vi "getData.vi"(8 "error in (no error)":errorcluster, 10 "device_name":string, 11 "ScriptEventList in":refnum<class "ScriptEventList.lvclass">) -> (0 "error out":errorcluster, 1 "singleToneData":T2(array[cluster]), 2 "data out":T3(array[cluster]) {"time" format="%_18g"}, 3 "ScriptEventList out":refnum<class "ScriptEventList.lvclass">, 4 "dataType":T1(ring))   [LabVIEW 2011, in "Tools.lvlib" / "Scripting.lvlib" / "ScriptEventList.lvclass"]
uses:
  ScriptEventList.lvclass
  DatabaseHelpers/Database Objects/Channel/Channel.lvclass
  ScriptEventList.lvclass/ScriptEventList.ctl
  ScriptEvent.lvclass
  ScriptEvents/SingleTone/SingleTone.lvclass
panel:
  out "Array":dbl[](array[numeric]) format="%_10g"
  out "times out":dbl[](array[numeric]) format="%_10g"
  out "appended array":dbl[](array[numeric]) format="%_13g"
  out "out":dbl[](array[numeric]) format="%_18g"
  out "in":dbl[](array[numeric])
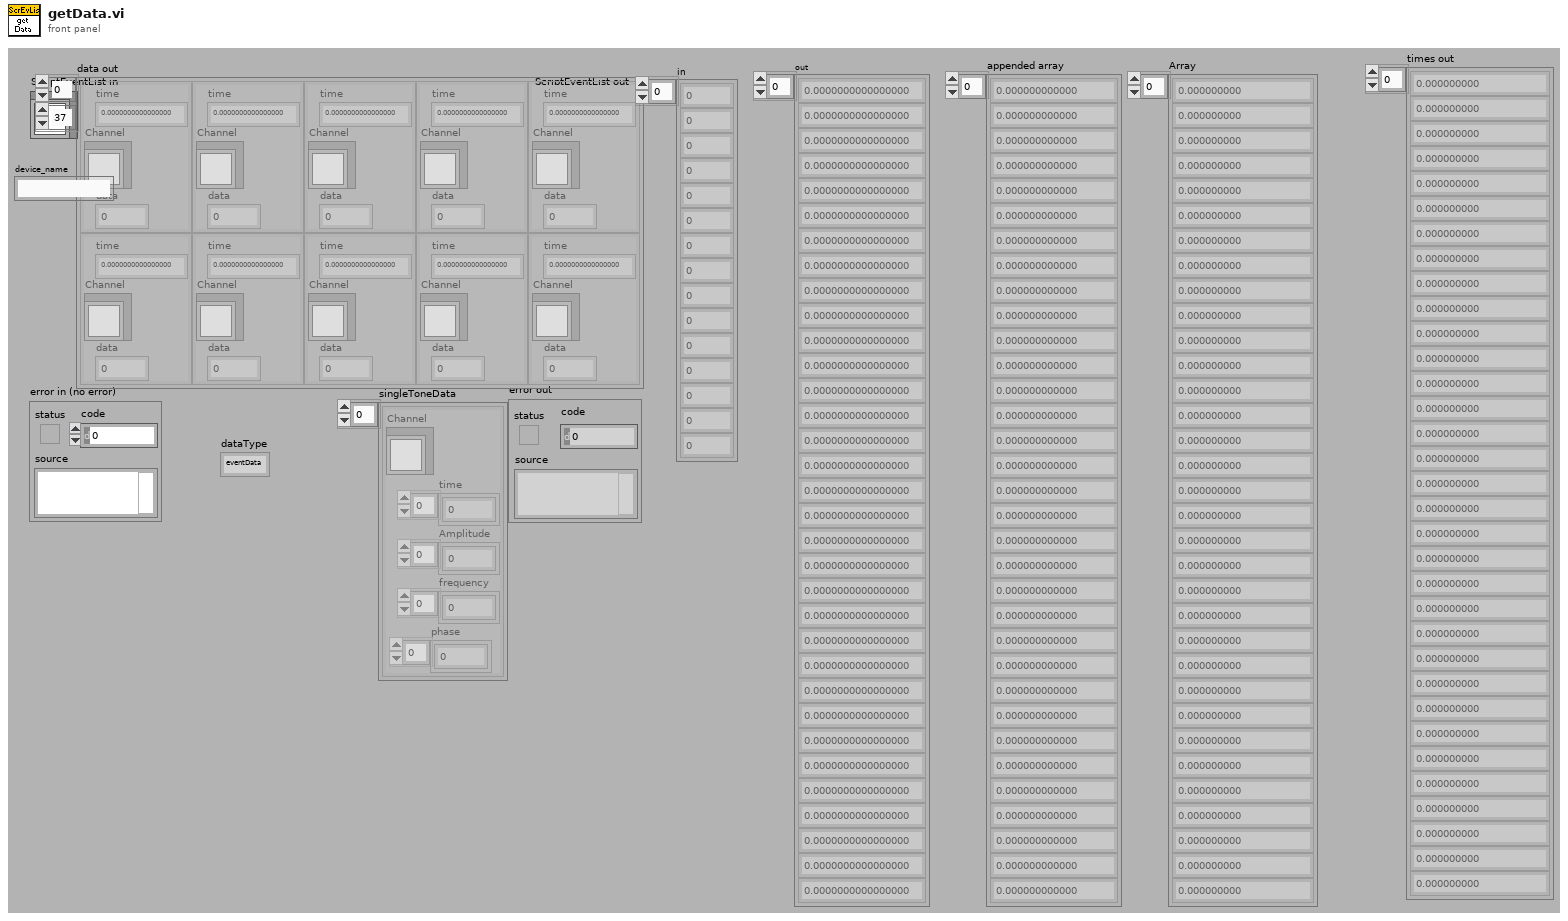
[diagram p1: front panel]
types:
  T1 = enum16{"eventData", "singleToneData", "fileData"}
  T2 = cluster{"Channel":refnum<class "Channel.lvclass">, "time":dbl[], "Amplitude":dbl[], "frequency":dbl[], "phase":dbl[]}[]
  T3 = cluster{"time":dbl, "Channel":refnum<class "Channel.lvclass">, "data":dbl}[][]
  T4 = cluster{"times":dbl[], "Channel":refnum<class "Channel.lvclass">, "data":dbl[]}
  T5 = cluster{"Tools.lvlib:DatabaseHelpers.lvlib:Channel.lvclass":refnum<class "Channel.lvclass">, "time":dbl[], "Amplitude":dbl[], "frequency":dbl[], "phase":dbl[]}[]
  T6 = cluster{dbl, "Channel":refnum<class "Channel.lvclass">, dbl}[][]
  T7 = cluster{"time":dbl, "Channel":refnum<class "Channel.lvclass">, "value":dbl}[][]
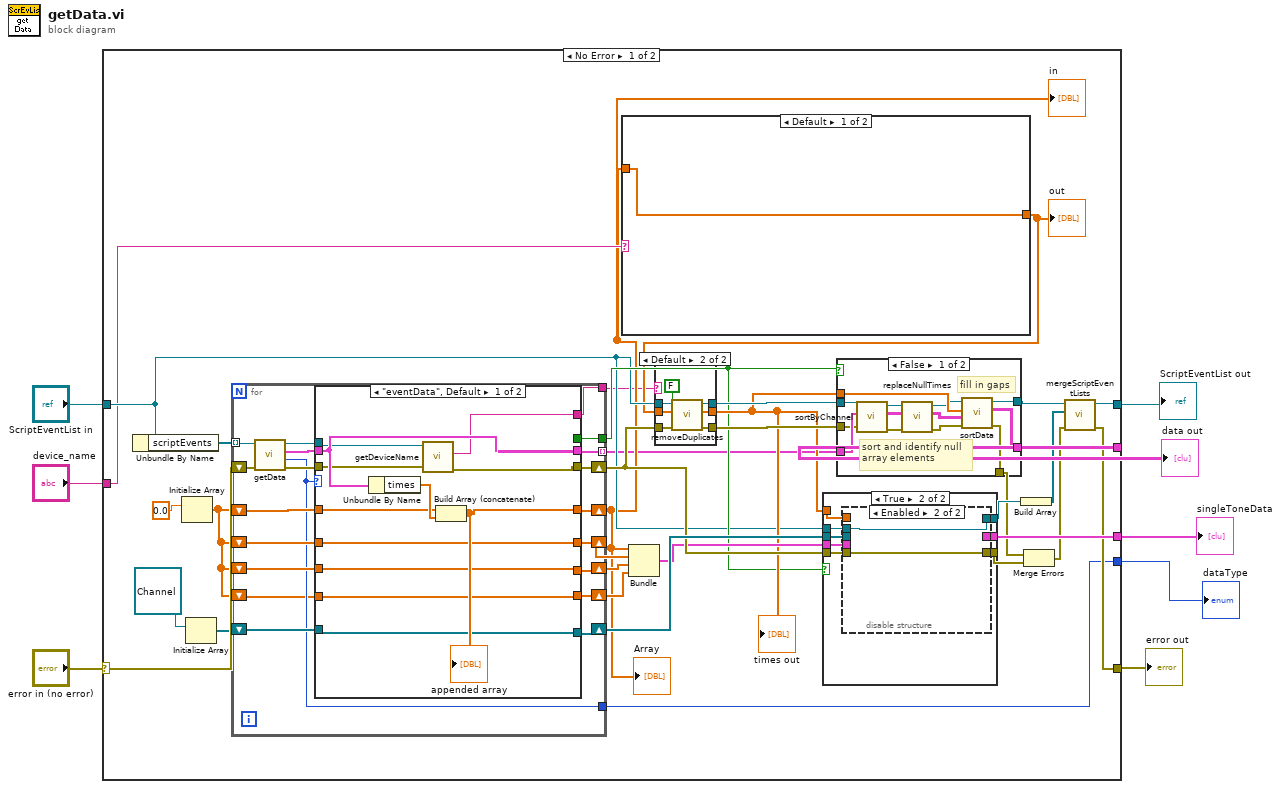
[diagram p0: block diagram]
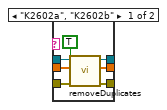
[diagram p2: hidden frame]
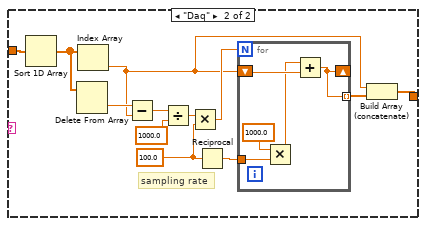
[diagram p3: hidden frame]
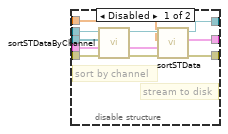
[diagram p5: hidden frame]
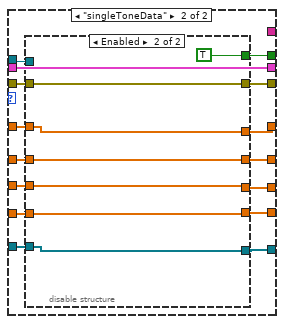
[diagram p7: hidden frame]
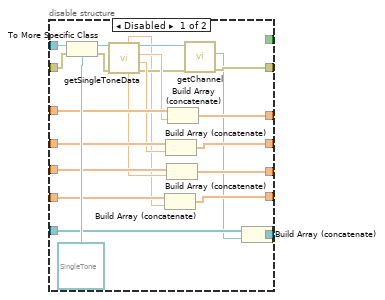
[diagram p8: hidden frame]
diagram:
  n1 = case shown="No Error" "error in (no error)" {
    selector: "error in (no error)" -> [w40 w190]
    tunnel: [w18 w190] -> w7
    tunnel: [w24 w189] -> w5
    tunnel: "ScriptEventList in" -> [w14 w189]
    tunnel: [w37 _] -> w4
    tunnel: [w27 _] -> w3
    tunnel: [w17 _] -> w2
    tunnel: "device_name" -> [w13 _]
    frame No Error {
      n2 = Unbundle By Name(w14) -> ("scriptEvents"=w41:refnum<class "ScriptEvent.lvclass">[])
      n3 = Initialize Array(0.0) -> (w16:dbl[])  [unwired: 1 in]
      n4 = Initialize Array(refnum<class "Channel.lvclass"> refnum ("Tools.lvlib:DatabaseHelpers.lvlib:Channel.lvclass")) -> (w34:refnum<class "Channel.lvclass">[])  [unwired: 1 in]
      n5 = for {
        tunnel: w41 -> [w131] mode=indexing
        shift-right: [w124] -> w31
        shift-left: w40 -> [w130]
        tunnel: [w126] -> w10 mode=indexing
        shift-right: [w128] -> w12
        shift-left: w16 -> [w129]
        shift-right: [w121] -> w33
        shift-left: w16 -> [w122]
        shift-right: [w120] -> w28
        shift-left: w16 -> [w119]
        shift-right: [w117] -> w32
        shift-left: w34 -> [w118]
        tunnel: [w116] -> w26
        tunnel: [w115] -> w17
        shift-right: [w113] -> w15
        shift-left: w16 -> [w114]
        tunnel: [w112] -> w9
        n6 = call-dynamic "getData.vi"("error in (no error)"=w130, "ScriptEvent in"=w131) -> ("error out"=w125:errorcluster, "dataType"=w115:T1, "data"=w127:T4, "ScriptEvent out"=w123:refnum<class "ScriptEvent.lvclass">)  [unwired: 6 in]
        n7 = case shown="\"eventData\", Default" w115 {
          tunnel: w129 -> [w142 w156]
          tunnel: [w141 w157] -> w128
          tunnel: w127 -> [w140 w144]
          tunnel: [w140 w144] -> w126
          tunnel: w125 -> [w134 w155]
          tunnel: [w133 w150] -> w124
          tunnel: w123 -> [w135 w158]
          tunnel: w122 -> [w139 w154]
          tunnel: [w139 w153] -> w121
          tunnel: [w138 w152] -> w120
          tunnel: w119 -> [w138 w151]
          tunnel: w118 -> [w136 w149]
          tunnel: [w136 w148] -> w117
          tunnel: [_ w147] -> w116
          tunnel: w114 -> [w137 w146]
          tunnel: [w137 w145] -> w113
          tunnel: [w132 _] -> w112
          frame "eventData", Default {
            n8 = Unbundle By Name(w140) -> ("times"=w143:dbl[])
            n9 = call "getDeviceName.vi"("error in (no error)"=w134, "ScriptEvent in"=w135) -> ("error out"=w133:errorcluster, "deviceName"=w132:string)  [unwired: 7 in, 1 out]
            n10 = Build Array (concatenate)(w142, w143) -> (w141:dbl[])
            "appended array" <- w141
          }
          frame "singleToneData" {
            n11 = disable-structure shown="Enabled" {
              disable-tunnel: w158 -> [w181 _]
              disable-tunnel: [w177 w187] -> w157
              disable-tunnel: w156 -> [w176 w187]
              disable-tunnel: w155 -> [w174 w183]
              disable-tunnel: w154 -> [w173 w186]
              disable-tunnel: [w172 w186] -> w153
              disable-tunnel: [w170 w185] -> w152
              disable-tunnel: w151 -> [w169 w185]
              disable-tunnel: [w165 w183] -> w150
              disable-tunnel: w149 -> [w164 w182]
              disable-tunnel: [w163 w182] -> w148
              disable-tunnel: [_ TRUE] -> w147
              disable-tunnel: w146 -> [w162 w184]
              disable-tunnel: [w161 w184] -> w145
              frame Disabled {
                n12 = To More Specific Class(target class=refnum<class "SingleTone.lvclass"> refnum ("Tools.lvlib:Scripting.lvlib:SingleTone.lvclass"), reference=w181, error in=w174) -> (specific class reference=w179:refnum<class "SingleTone.lvclass">, error out=w178:errorcluster)
                n13 = call "getSingleToneData.vi"("error in (no error)"=w178, "SingleTone in"=w179) -> ("error out"=w166:errorcluster, "amplitude"=w171:dbl, "time"=w175:dbl, "SingleTone out"=w167:refnum<class "SingleTone.lvclass">, "frequency"=w168:dbl, "phase"=w160:dbl)  [unwired: 4 in]
                n14 = Build Array (concatenate)(w162, w160) -> (w161:dbl[])
                n15 = Build Array (concatenate)(w173, w171) -> (w172:dbl[])
                n16 = Build Array (concatenate)(w169, w168) -> (w170:dbl[])
                n17 = Build Array (concatenate)(w176, w175) -> (w177:dbl[])
                n18 = call-dynamic "getChannel.vi"("error in (no error)"=w166, "ScriptEvent.lvclass in"=w167) -> ("error out"=w165:errorcluster, "Channel.lvclass"=w159:refnum<class "Channel.lvclass">)  [unwired: 7 in, 1 out]
                n19 = Build Array (concatenate)(w164, w159) -> (w163:refnum<class "Channel.lvclass">[])
              }
              frame Enabled {
              }
            }
          }
        }
      }
      "in" <- w12
      "Array" <- w12
      n20 = case shown="Default" w13 {
        tunnel: [w56 w58] -> w11
        tunnel: w12 -> [w56 w60]
        frame Default {
        }
        frame "Daq" {
          w63 = 100.0
          # "sampling rate"
          n21 = Sort 1D Array(array=w60) -> (sorted array=w68:dbl[])
          n22 = Delete From Array(array=w68) -> (deleted portion=w67:dbl)  [unwired: 2 in, 1 out]
          n23 = Index Array(array=w68) -> (element=w57:dbl)  [unwired: 1 in]
          n24 = Subtract(x=w67, y=w57) -> (x-y=w66:dbl)
          n25 = Divide(x=w66, y=1000.0) -> (x/y=w64:dbl)
          n26 = Multiply(x=w64, y=w63) -> (x*y=w61:dbl)
          n27 = Reciprocal(x=w63) -> (1/x=w62:dbl)
          n28 = for {
            N: w61 -> [_]
            tunnel: w62 -> [w72]
            tunnel: [w69] -> w59 mode=indexing
            shift-right: [w69] -> _
            shift-left: w57 -> [w73]
            n29 = Multiply(x=1000.0, y=w72) -> (x*y=w70:dbl)
            n30 = Add(x=w70, y=w73) -> (x+y=w69:dbl)
          }
          n31 = Build Array (concatenate)(w57, w59) -> (w58:dbl[])
        }
      }
      "out" <- w11
      n32 = Bundle(w12, w33, w28, w15) -> (w30:cluster{dbl[], dbl[], dbl[], dbl[]})  [unwired: 1 in]
      n33 = case shown="Default" w9 {
        tunnel: [w48 w55] -> w38
        tunnel: [w47 w54] -> w36
        tunnel: w31 -> [w46 w53]
        tunnel: [w45 w52] -> w29
        tunnel: w14 -> [w44 w51]
        tunnel: w11 -> [w43 w50]
        frame "K2602a", "K2602b" {
          n34 = call "removeDuplicates.vi"("error in (no error)"=w46, "Don't add t zero"=TRUE, "times"=w43, "ScriptEventList in"=w44) -> ("error out"=w47:errorcluster, "times out"=w45:dbl[], "ScriptEventList out"=w48:refnum<class "ScriptEventList.lvclass">)  [unwired: 5 in]
        }
        frame Default {
          n35 = call "removeDuplicates.vi"("error in (no error)"=w53, "Don't add t zero"=FALSE, "times"=w50, "ScriptEventList in"=w51) -> ("error out"=w54:errorcluster, "times out"=w52:dbl[], "ScriptEventList out"=w55:refnum<class "ScriptEventList.lvclass">)  [unwired: 5 in]
        }
      }
      "times out" <- w29
      n36 = case shown="True" w26 {
        tunnel: w14 -> [w75 w83]
        tunnel: w32 -> [_ w82]
        tunnel: w31 -> [w74 w81]
        tunnel: w30 -> [_ w80]
        tunnel: w29 -> [_ w79]
        tunnel: [_ w78] -> w27
        tunnel: [w75 w77] -> w23
        tunnel: [w74 w76] -> w20
        frame False {
        }
        frame True {
          n37 = disable-structure shown="Enabled" {
            disable-tunnel: w83 -> [w94 w95]
            disable-tunnel: w82 -> [w93 _]
            disable-tunnel: w81 -> [w92 w96]
            disable-tunnel: w80 -> [w91 _]
            disable-tunnel: w79 -> [w88 _]
            disable-tunnel: [w86 _] -> w78
            disable-tunnel: [w85 w95] -> w77
            disable-tunnel: [w84 w96] -> w76
            frame Disabled {
              # "stream to disk"
              # "sort by channel"
              n38 = call "sortSTDataByChannel.vi"("error in (no error)"=w92, "data"=w91, "channels"=w93, "ScriptEventList in"=w94) -> ("error out"=w87:errorcluster, "channelData"=w89:T5, "ScriptEventList out"=w90:refnum<class "ScriptEventList.lvclass">)  [unwired: 5 in]
              n39 = call "sortSTData.vi"("error in (no error)"=w87, "channelData"=w89, "times"=w88, "ScriptEventList in"=w90) -> ("error out"=w84:errorcluster, "sortedData"=w86:T2, "ScriptEventList out"=w85:refnum<class "ScriptEventList.lvclass">)  [unwired: 5 in]
            }
            frame Enabled {
            }
          }
        }
      }
      n40 = case shown="False" w26 {
        tunnel: [w109 w111] -> w25
        tunnel: w38 -> [w108 w111]
        tunnel: w10 -> [w107 _]
        tunnel: [w106 _] -> w37
        tunnel: w36 -> [w105 w110]
        tunnel: [w104 w110] -> w21
        tunnel: w29 -> [w103 _]
        frame False {
          # "fill in gaps"
          # "sort and identify null\narray elements"
          n41 = call "sortByChannel.vi"("error in (no error)"=w105, "Array"=w107, "ScriptEventList in"=w108) -> ("error out"=w98:errorcluster, "data"=w102:T6, "ScriptEventList out"=w100:refnum<class "ScriptEventList.lvclass">)  [unwired: 6 in]
          n42 = call "replaceNullTimes.vi"("error in (no error)"=w98, "data in"=w102, "ScriptEventList in"=w100) -> ("error out"=w97:errorcluster, "data out"=w101:T7, "ScriptEventList out"=w99:refnum<class "ScriptEventList.lvclass">)  [unwired: 6 in]
          n43 = call "sortData.vi"("error in (no error)"=w97, "data"=w101, "times"=w103, "ScriptEventList in"=w99) -> ("error out"=w104:errorcluster, "data out"=w106:T3, "ScriptEventList out"=w109:refnum<class "ScriptEventList.lvclass">)  [unwired: 5 in]
        }
        frame True {
        }
      }
      n44 = Build Array(w23) -> (w22:refnum<class "ScriptEventList.lvclass">[])
      n45 = Merge Errors(w21, w20) -> (w19:errorcluster)
      n46 = call "mergeScriptEventLists.vi"("error in (no error)"=w19, "Array"=w22, "ScriptEventList in"=w25) -> ("error out"=w18:errorcluster, "ScriptEventList out"=w24:refnum<class "ScriptEventList.lvclass">)  [unwired: 7 in]
    }
    frame Error {
    }
  }
  "error out" <- w7
  "ScriptEventList out" <- w5
  "data out" <- w4
  "singleToneData" <- w3
  "dataType" <- w2
